vi "readFromXML.vi"(8 "error in (no error)":errorcluster, 10 "XML in":string, 11 "CollimationOffsetCommands in":refnum<class "CollimationOffsetCommands.lvclass">) -> (0 "error out":errorcluster, 3 "CollimationOffsetCommands out":refnum<class "CollimationOffsetCommands.lvclass">)   [LabVIEW 2022 SP3, in "TCSDataDefinitions.lvlib" / "TCSCommand.lvlib" / "OffsetCommands.lvlib" / "CollimationOffsetCommands.lvclass"]
uses:
  CollimationOffsetCommands.lvclass
  OffsetCommands/OffsetCommands.lvclass
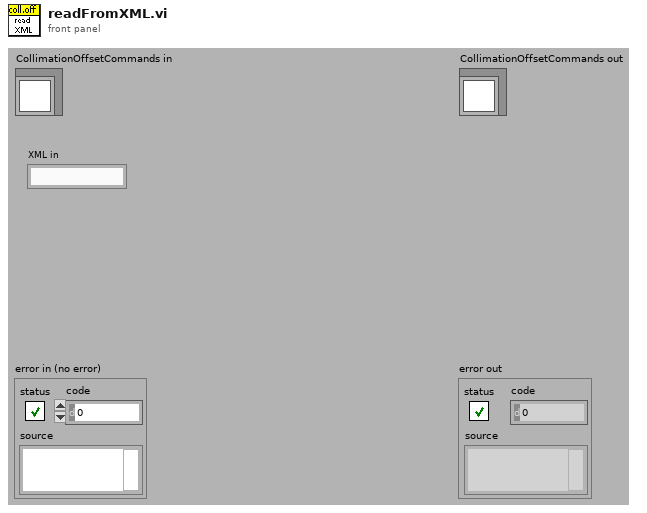
[diagram p1: front panel]
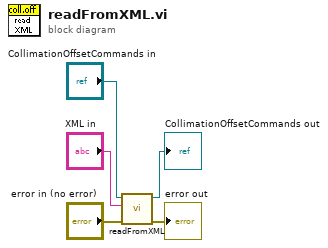
[diagram p0: block diagram]
diagram:
  n1 = call-parent "readFromXML.vi"("error in (no error)"="error in (no error)", "XML in"="XML in", "OffsetCommands in"="CollimationOffsetCommands in") -> ("error out"=→"error out":errorcluster, "OffsetCommands out"=→"CollimationOffsetCommands out":refnum<class "CollimationOffsetCommands.lvclass">)  [unwired: 7 out]
